vi "Apply.vi"(8 "error in":errorcluster, 11 "DIO DAQmx PWM CFG in":refnum<class "CO DAQmx PWM CFG Simulated.lvclass">) -> (0 "error out":errorcluster, 3 "DIO DAQmx PWM CFG out":refnum<class "CO DAQmx PWM CFG Simulated.lvclass">)   [LabVIEW 2024, in "DAQmx Simulated CFGs.lvlib" / "CO DAQmx PWM CFG Simulated.lvclass"]
uses:
  CO DAQmx PWM CFG Simulated.lvclass
  Configurations/CFG Base/CFG Base.lvclass/CFG Base.ctl
  CO DAQmx PWM CFG/CO DAQmx PWM CFG.lvclass
  Configurations/CFG Base/CFG Base.lvclass
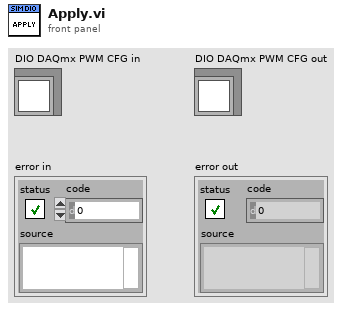
[diagram p1: front panel]
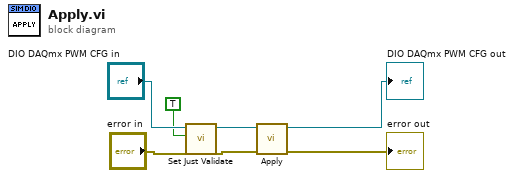
[diagram p0: block diagram]
diagram:
  n1 = call "Set Just Validate.vi"("Just Validate"=TRUE, "CFG Base in"="DIO DAQmx PWM CFG in") -> ("CFG Base out"=w3:refnum<class "CO DAQmx PWM CFG Simulated.lvclass">)  [unwired: 9 in]
  n2 = call-parent "Apply.vi"("error in (no error)"="error in", "DIO DAQmx PWM CFG in"=w3) -> ("error out"=→"error out":errorcluster, "DIO DAQmx PWM CFG out"=→"DIO DAQmx PWM CFG out":refnum<class "CO DAQmx PWM CFG Simulated.lvclass">)  [unwired: 8 in]
